vi "Vision Scaling file Read write.vi"(7 "Enum":enum16{"Write", "Read"}(ring), 8 "error in (no error)":errorcluster, 9 "all rows":string[][](array[string]), 10 "dup path":path, 11 "Vision tool":string) -> (0 "error out":errorcluster, 3 "all rows":string[][](array[string]))   [LabVIEW 2020]
uses:
  <vilib>/Utility/file.llb/Write Delimited Spreadsheet (string).vi
  <vilib>/Utility/file.llb/Read Delimited Spreadsheet (string).vi
panel:
  out "file or folder exists?":bool
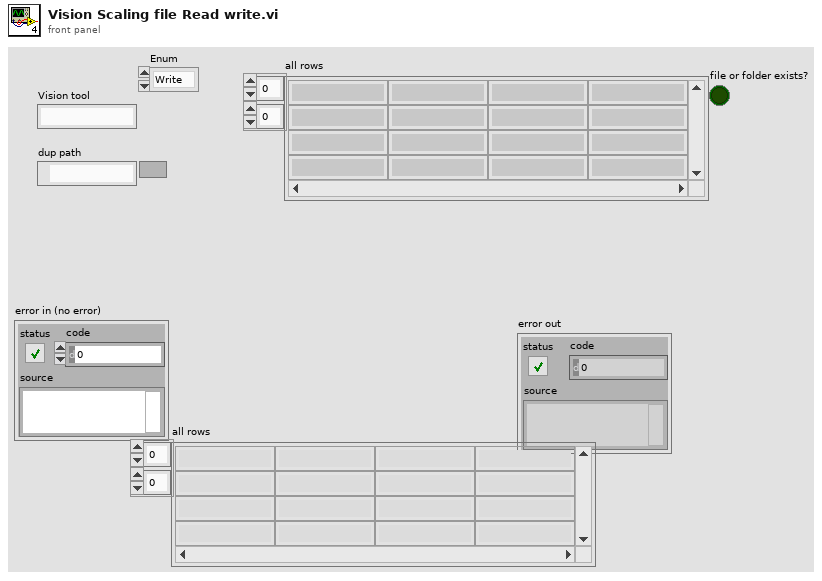
[diagram p1: front panel]
types:
  T1 = enum16{"open", "replace", "create", "open or create", "replace or create", "replace or create with confirmation"}
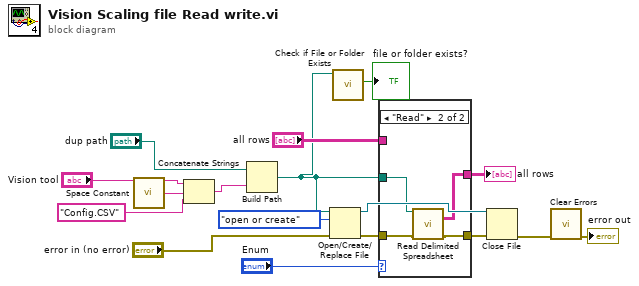
[diagram p0: block diagram]
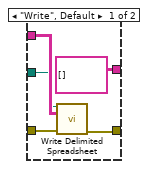
[diagram p2: hidden frame]
diagram:
  n1 = call <vilib>:"Space Constant.vi"() -> ("String"=w14:string)
  n2 = Concatenate Strings("Vision tool", w14, "Config.CSV" ("string")) -> (w17:string)
  n3 = Build Path(base path="dup path", name or relative path=w17) -> (appended path=w2:path)
  n4 = Open/Create/Replace File(file path (use dialog)=w2, error in="error in (no error)", operation (0:open)=T1."open or create") -> (refnum out=w11:refnum<file>, error out=w10:errorcluster)  [unwired: 3 in, 1 out]
  n5 = call <vilib>:"Check if File or Folder Exists.vi"("path"=w2) -> ("file or folder exists?"=→"file or folder exists?":bool)  [unwired: 8 in, 2 out]
  n6 = case shown="\"Read\"" "Enum" {
    tunnel: w2 -> [w18 w26]
    tunnel: w10 -> [w22 w25]
    tunnel: [w21 w24] -> w9
    tunnel: [string[][] [] ("all rows") w23] -> w8
    tunnel: "all rows" -> [w20 _]
    frame "Write", Default {
      n7 = call-poly <vilib>:"Write Delimited Spreadsheet.vi"("file path (dialog if empty)"=w18, "2D data"=w20, "error in (no error)"=w22) -> ("error out"=w21:errorcluster)  [unwired: 11 in, 1 out]
    }
    frame "Read" {
      n8 = call-poly <vilib>:"Read Delimited Spreadsheet.vi"("file path (dialog if empty)"=w26, "error in (no error)"=w25) -> ("all rows"=w23:string[][], "error out"=w24:errorcluster)  [unwired: 8 in, 4 out]
    }
  }
  "all rows" <- w8
  n9 = Close File(refnum=w11, error in=w9) -> (error out=w4:errorcluster)  [unwired: 1 out]
  n10 = call <vilib>:"Clear Errors.vi"("error in (no error)"=w4) -> ("error out"=→"error out":errorcluster)  [unwired: 5 in, 1 out]
